vi "addTemperature.vi"(8 "error in (no error)":errorcluster, 10 "lastTempMeasure":dbl, 11 "State in":refnum<class "ElectrometerState.lvclass">) -> (0 "error out":errorcluster, 3 "State out":refnum<class "ElectrometerState.lvclass">)   [LabVIEW 2016]
uses:
  ElectrometerState.lvclass
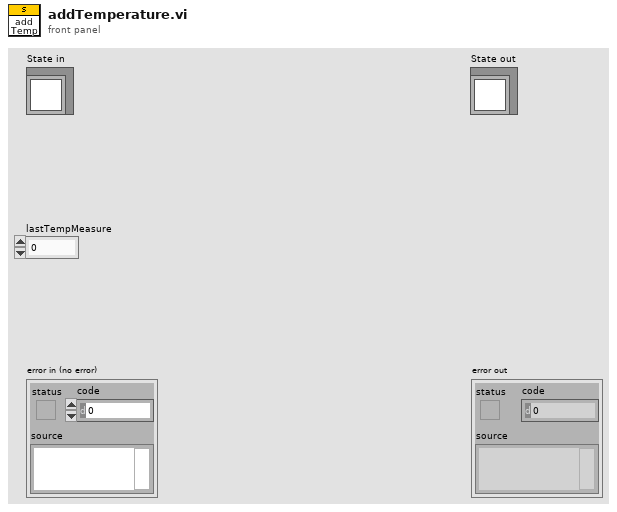
[diagram p1: front panel]
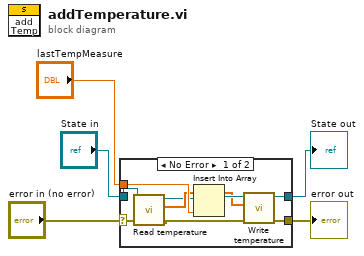
[diagram p0: block diagram]
diagram:
  n1 = case shown="No Error" "error in (no error)" {
    selector: "error in (no error)" -> [w12 w16]
    tunnel: [w9 w16] -> w4
    tunnel: [w10 w15] -> w2
    tunnel: "State in" -> [w13 w15]
    tunnel: "lastTempMeasure" -> [w14 _]
    frame No Error {
      n2 = call-dynamic "Read temperature.vi"("error in (no error)"=w12, "ElectrometerState in"=w13) -> ("error out"=w8:errorcluster, "temperature"=w11:dbl[], "ElectrometerState out"=w7:refnum<class "ElectrometerState.lvclass">)  [unwired: 7 in]
      n3 = Insert Into Array(array=w11, new element=w14) -> (w6:dbl[])  [unwired: 1 in]
      n4 = call-dynamic "Write temperature.vi"("error in (no error)"=w8, "temperature"=w6, "ElectrometerState in"=w7) -> ("error out"=w9:errorcluster, "ElectrometerState out"=w10:refnum<class "ElectrometerState.lvclass">)  [unwired: 7 in]
    }
    frame Error {
    }
  }
  "error out" <- w4
  "State out" <- w2
